vi "Constants.vi"() -> ()   [LabVIEW 2018]
panel:
  in  "4bar Cargo Ship Ball":dbl=1700.0
  in  "4bar Cargo Ship Hatch":dbl=375.0
  in  "4barMotionMagic":T1={"Cruise Velocity"=450, "Acceleration"=250}
  in  "HPIntakePositionPIDF":T2={"P"=3.0, "I"=0.0, "D"=300.0, "F"=0.0, "I Zone"=0.0}
  in  "4barPositionPIDF":T2={"P"=5.0, "I"=0.0, "D"=70.0, "F"=0.07, "I Zone"=0.0}
  in  "Gyro Angle \"Calibration\" Proportion":dbl
  in  "Drive Allowable Error":dbl=150.0
  in  "4bar horizantal position kF":dbl
  in  "4bar Encoder to Angle Ratio":dbl
  in  "Encoder Counts Per Rotation":dbl=4096.0
  in  "Wheel Diameter":dbl=6.0
  in  "HP Intake Wall":dbl=-2350.0
  in  "HP Intake Floor":dbl=-1750.0
  in  "HP Intake Home":dbl
  in  "RightDriveMotionMagic":T1={"Cruise Velocity"=3500, "Acceleration"=750}
  in  "LeftDriveMotionMagic":T1={"Cruise Velocity"=3500, "Acceleration"=750}
  in  "4bar Bottom Position":dbl=175.0
  in  "4bar Low Position":dbl=1100.0
  in  "4bar Mid Position":dbl=2200.0
  in  "4bar High Position":dbl=3500.0
  in  "RightDrivePositionPIDF":T2={"P"=2.5, "I"=0.0, "D"=180.0, "F"=0.04, "I Zone"=0.0}
  in  "LeftDrivePositionPIDF":T2={"P"=3.5, "I"=0.0, "D"=180.0, "F"=0.04, "I Zone"=0.0}
  in  "Cargo Open Ramp":dbl=0.3
  in  "4bar Ramp":dbl=0.2
  in  "Drive Closed Loop Ramp":dbl=0.5
  in  "Drive Open Loop Ramp":dbl=0.5
  # "Intake STUFF"
  # "4bar STUFF"
  # "DRIVE STUFF"
  # "Make this F 0"
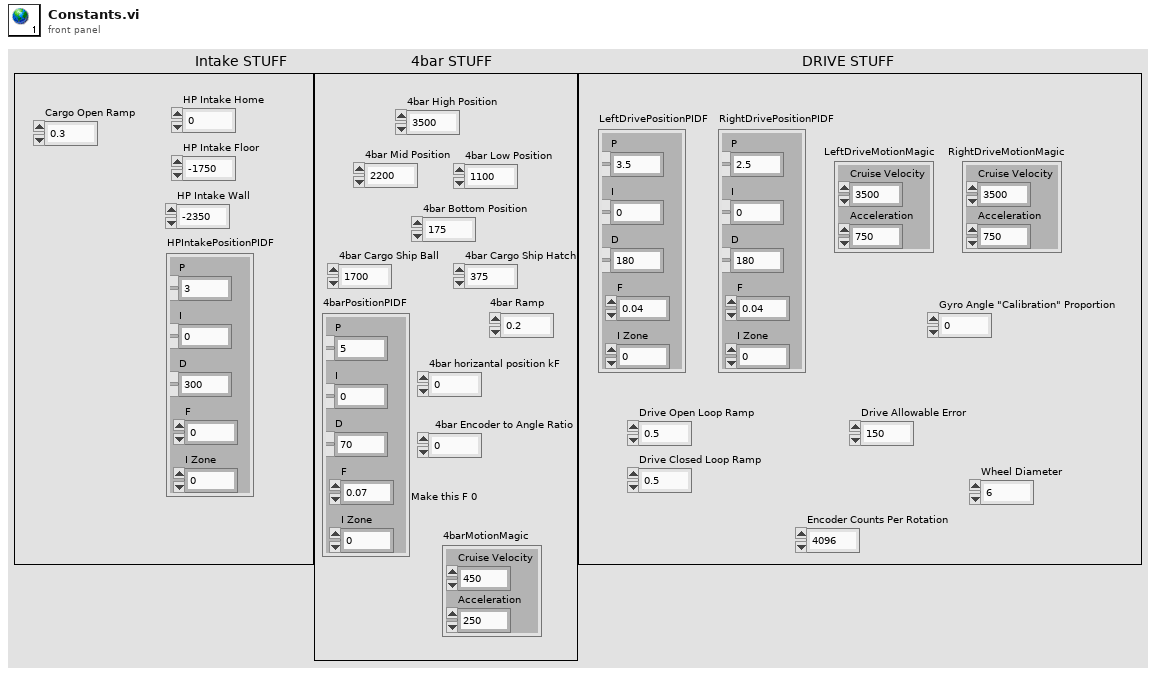
[diagram p1: front panel]
types:
  T1 = cluster{"Cruise Velocity":i32, "Acceleration":i32}
  T2 = cluster{"P":dbl, "I":dbl, "D":dbl, "F":dbl, "I Zone":dbl}
diagram:
